vi "MakeWall.vi"(8 "error in (no error)":errorcluster, 11 "BombedMazeGame":refnum<class "BombedMazeGame.lvclass">) -> (0 "error out":errorcluster, 2 "Wall":refnum<class "Wall.lvclass">, 3 "BombedMazeGame":refnum<class "BombedMazeGame.lvclass">)   [LabVIEW 2020, in "FactoryMethod.lvlib" / "NoParametrizedFactoryMethod.lvlib" / "BombedMazeGame.lvclass"]
uses:
  BombedMazeGame.lvclass
  GoFcommonClasses/ConcreteMazeSite/Wall/Wall.lvclass
  GoFcommonClasses/ConcreteMazeSite/BombedWall/BombedWall.lvclass
  E:/Francesco/GitHub/Design-Patterns-GoF_-_NI-LV/Creational/GoFcommonClasses/ConcreteMazeSite/Wall/Wall.lvclass
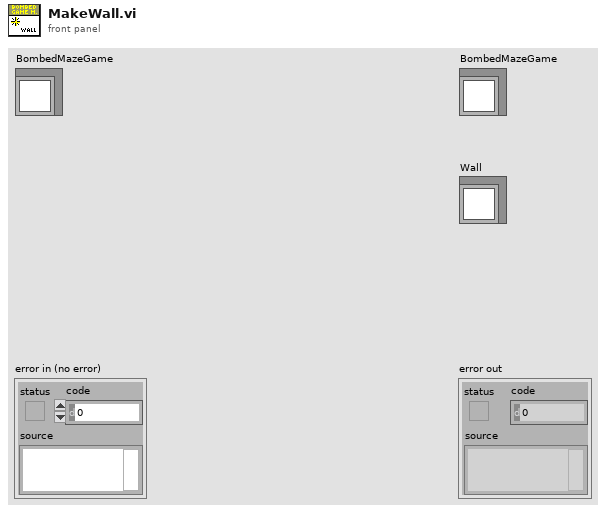
[diagram p1: front panel]
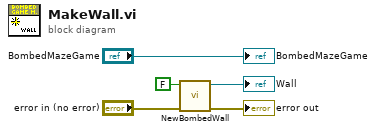
[diagram p0: block diagram]
diagram:
  n1 = call "NewBombedWall.vi"("error in (no error)"="error in (no error)", "Bomb"=FALSE) -> ("error out"=→"error out":errorcluster, "BombedWall"=→"Wall":refnum<class "BombedWall.lvclass">)  [unwired: 8 in]
  "BombedMazeGame" <- "BombedMazeGame"
